vi "ROS_Topic_Write_Stop_Continuous_Primitive.vi"(3 "ROS in":T1={"topic port"=0, "Node"="", "topic"="", "type"="", "node port"=0, "error "={"status"=FALSE, "code"=0, "source"=""}, "Direction"=enum."Node", "APIs"=[], "Update (ms)"=1, "write queue"=1}) -> (1 "ROS out":T1={"topic port"=0, "Node"="", "topic"="", "type"="", "node port"=0, "error "={"status"=FALSE, "code"=0, "source"=""}, "Direction"=enum."Node", "APIs"=[], "Update (ms)"=1, "write queue"=1})   [LabVIEW 2010]
doc: "Instructs the server to stop publishing messages continuously."
uses:
  <userlib>/ROSforLV/ROS/Code/SubVIs/_ROSControl.ctl
  <userlib>/ROSforLV/ROS/Code/SubVIs/_ROSDirection.ctl
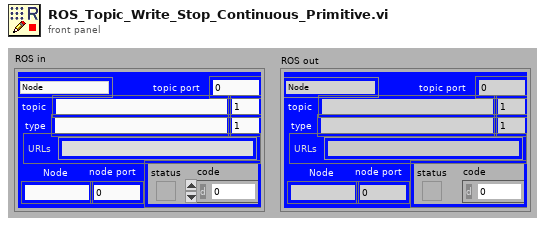
[diagram p1: front panel]
types:
  T1 = typedef "_ROSControl.ctl" = cluster{"topic port":u16, "Node":string, "topic":string, "type":string, "node port":u32, "error ":errorcluster, "Direction":T2, "APIs":string[], "Update (ms)":u16, "write queue":u16}
  T2 = typedef "_ROSDirection.ctl" = enum16{"Node", "Publisher", "Subscriber", "Service Client"}
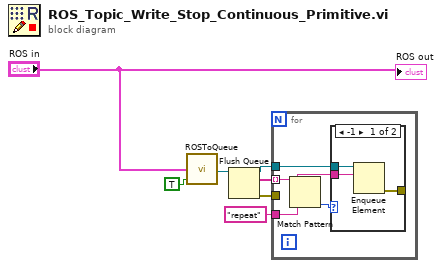
[diagram p0: block diagram]
diagram:
  n1 = call <userlib>:"ROSToQueue.vi"("Wait?"=TRUE, "ROS"="ROS in") -> ("queue"=w2:refnum<queue>)  [unwired: 2 in, 1 out]
  n2 = Flush Queue(queue=w2) -> (queue out=w3:refnum<queue>, remaining elements=w5:string[], error out=w1:errorcluster)  [unwired: 1 in]
  n3 = for {
    tunnel: w5 -> [w9] mode=indexing
    tunnel: "repeat" ("regular expression") -> [w11]
    tunnel: w3 -> [w8]
    tunnel: w1 -> [_]
    n4 = Match Pattern(string=w9, regular expression=w11) -> (offset past match=w10:i32)  [unwired: 1 in, 3 out]
    n5 = case shown="-1" w10 {
      tunnel: w9 -> [w14 _]
      tunnel: w8 -> [w13 _]
      tunnel: [w12 _] -> _
      frame -1 {
        n6 = Enqueue Element(queue=w13, element=w14) -> (error out=w12:errorcluster)  [unwired: 2 in, 2 out]
      }
      frame Default {
      }
    }
  }
  "ROS out" <- "ROS in"
